vi "arrange func.vi"(10 "input Parameter":T2={"input COP of ACs"=3.0, "input setDay Temp"=22.0, "input setNight Temp."=20.0}, 11 "input envTemp. & elecFee":cluster{"Temp.":dbl[], "elecFee":dbl[]}={"Temp."=[29.6, 26.5, 26.8, 26.8, 26.5, 26.9, 27.8, 28.5, 26.3, 30.1, 33.3, 33.4, 33.9, 32.2, 32.7, 32.7, 32.4, 31.5, 30.5, 29.7, 28.3, 28.2, 27.9, 27.5], "elecFee"=[2.2, 2.2, 2.2, 2.2, 2.2, 2.2, 2.2, 2.2, 3.5, 3.5, 3.5, 3.5, 3.5, 3.5, 3.5, 3.5, 3.5, 3.5, 3.5, 3.5, 3.5, 3.5, 2.2, 2.2]}) -> (0 "Outcome Total elecFee":dbl[](array[numeric]), 3 "OUTCOME":T1(array[cluster]))   [LabVIEW 2014]
panel:
  in  "group 3 power consume (W)":dbl format="%#_13g"
  in  "group 3 Lightening period (h)":i32
  in  "group 2 power consume (W)":dbl format="%#_13g"
  in  "group 2 Lightening period (h)":i32
  in  "group 1 power consume (W)":dbl format="%#_13g"
  in  "group 1 Lightening period (h)":i32
  in  "OK":bool
  # "0~1"
  # "1~2"
  # "2~3"
  # "3~4"
  # "4~5"
  # "5~6"
  # "6~7"
  # "7~8"
  # "8~98~9"
  # "9~10"
  # "10~11"
  # "11~12"
  # "12~13"
  # "13~14"
  # "14~15"
  # "15~16"
  # "16~17"
  # "17~18"
  # "18~19"
  # "19~20"
  # "21~21"
  # "21~22"
  # "22~23"
  # "23~24"
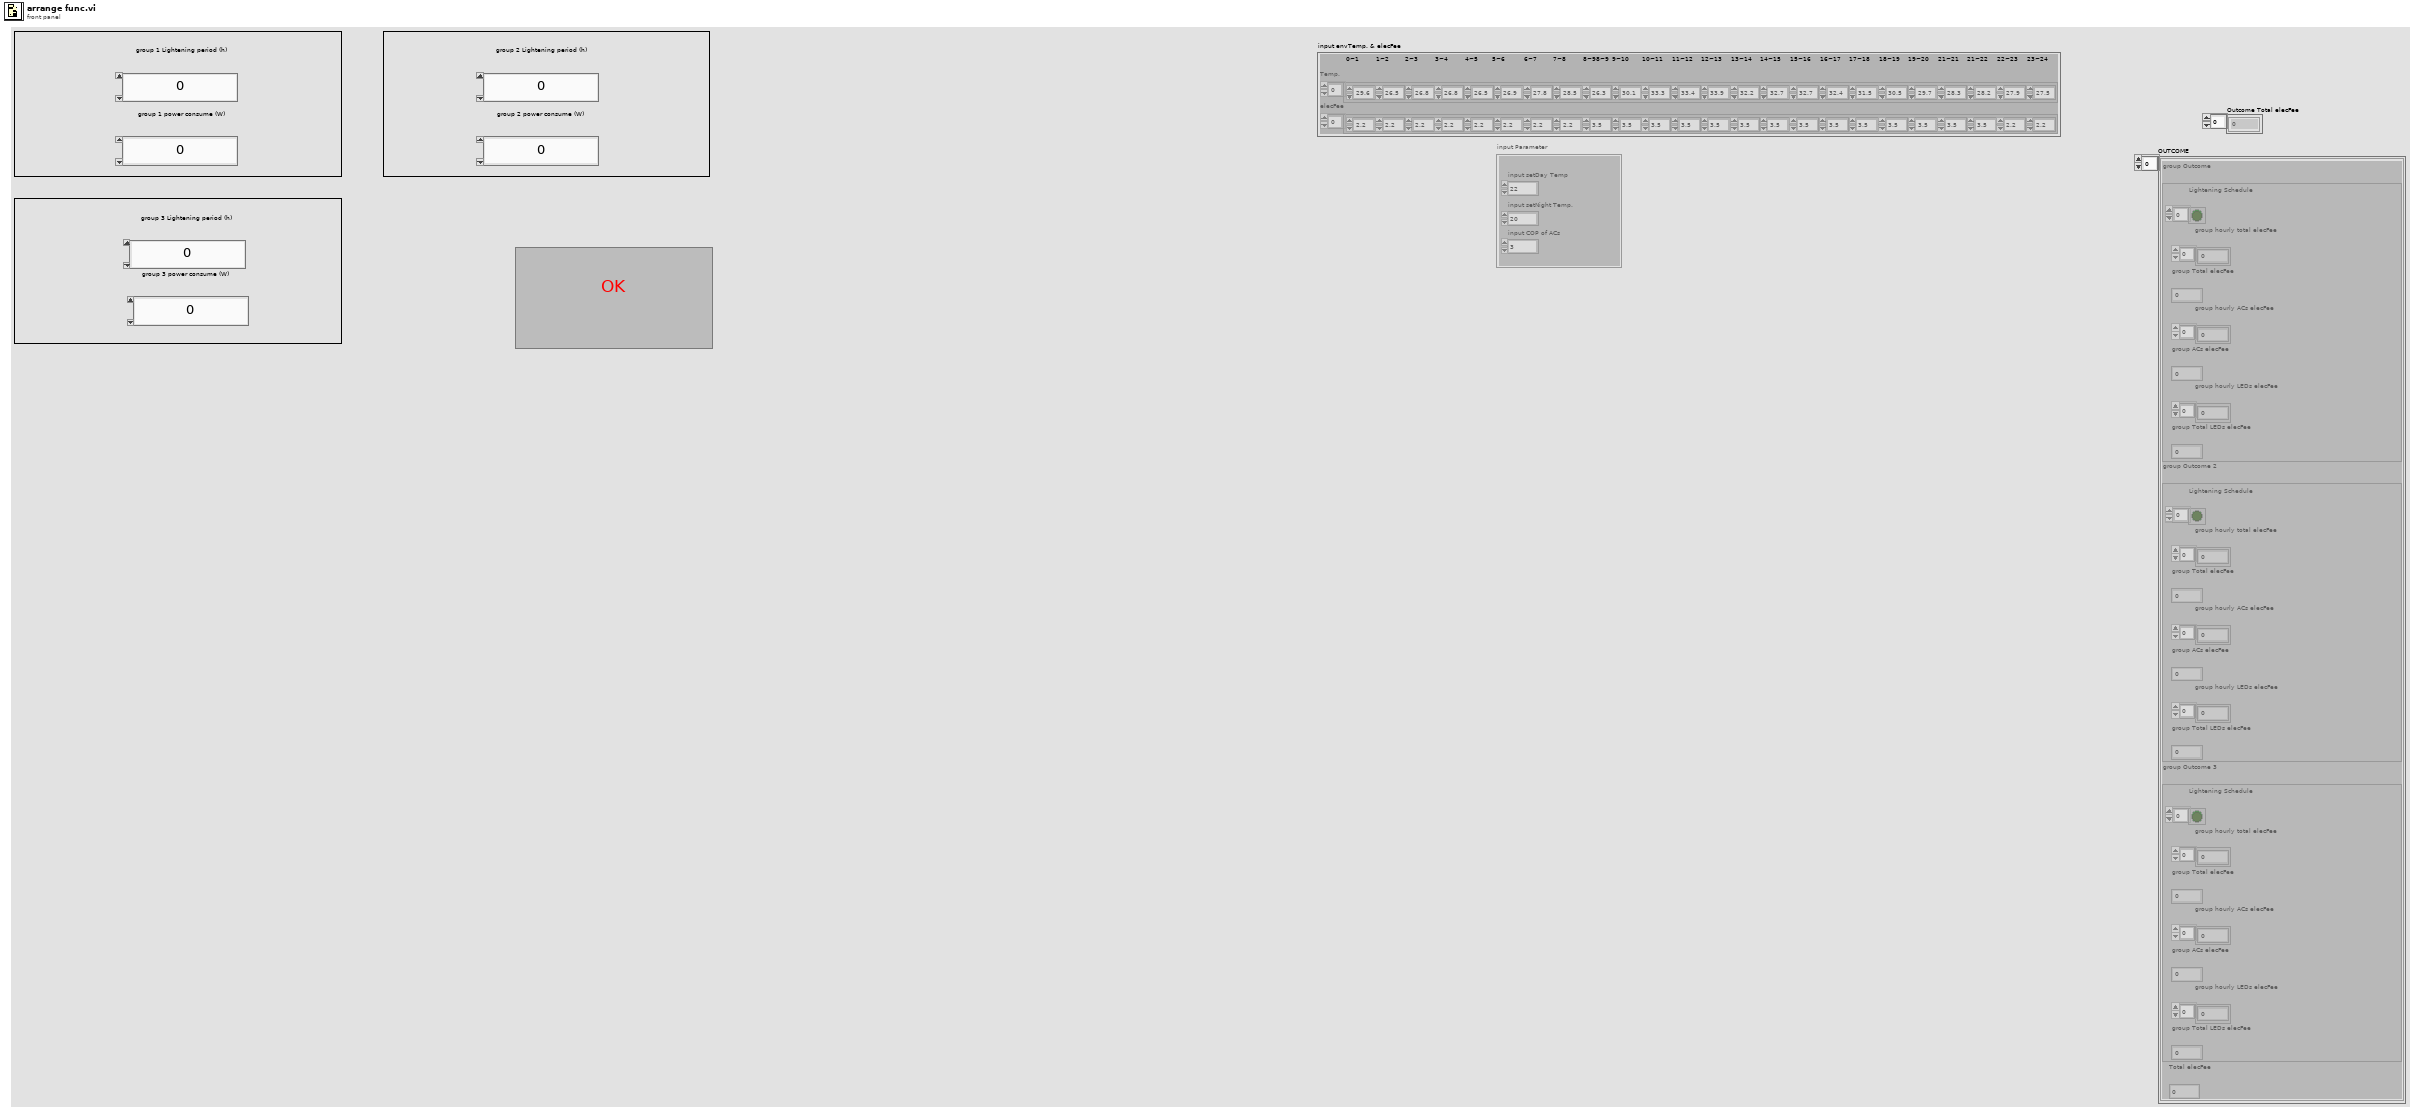
[diagram p1: front panel]
types:
  T1 = cluster{"group Outcome":cluster{"Lightening Schedule":bool[], "group hourly total elecFee":dbl[], "group Total elecFee":dbl, "group hourly ACs elecFee":dbl[], "group ACs elecFee":dbl, "group hourly LEDs elecFee":dbl[], "group Total LEDs elecFee":dbl}, "group Outcome 2":cluster{"Lightening Schedule":bool[], "group hourly total elecFee":dbl[], "group Total elecFee":dbl, "group hourly ACs elecFee":dbl[], "group ACs elecFee":dbl, "group hourly LEDs elecFee":dbl[], "group Total LEDs elecFee":dbl}, "group Outcome 3":cluster{"Lightening Schedule":bool[], "group hourly total elecFee":dbl[], "group Total elecFee":dbl, "group hourly ACs elecFee":dbl[], "group ACs elecFee":dbl, "group hourly LEDs elecFee":dbl[], "group Total LEDs elecFee":dbl}, "Total elecFee":dbl}[]
  T2 = cluster{"input COP of ACs":dbl, "input setDay Temp":dbl, "input setNight Temp.":dbl}
  T3 = cluster{"group Outcome":cluster{"Lightening Schedule":bool[], "group hourly total elecFee":dbl[], "group Total elecFee":dbl, "group hourly ACs elecFee":dbl[], "group ACs elecFee":dbl, "group hourly LEDs elecFee":dbl[], "group Total LEDs elecFee":dbl}, "group Outcome 2":cluster{"Lightening Schedule":bool[], "group hourly total elecFee":dbl[], "group Total elecFee":dbl, "group hourly ACs elecFee":dbl[], "group ACs elecFee":dbl, "group hourly LEDs elecFee":dbl[], "group Total LEDs elecFee":dbl}, "group Outcome 3":cluster{"Lightening Schedule":bool[], "group hourly total elecFee":dbl[], "group Total elecFee":dbl, "group hourly ACs elecFee":dbl[], "group ACs elecFee":dbl, "group hourly LEDs elecFee":dbl[], "group Total LEDs elecFee":dbl}, "Total elecFee":dbl}
  T4 = cluster{"Lightening Schedule":bool[], "group hourly total elecFee":dbl[], "group Total elecFee":dbl, "group hourly ACs elecFee":dbl[], "group ACs elecFee":dbl, "group hourly LEDs elecFee":dbl[], "group Total LEDs elecFee":dbl}
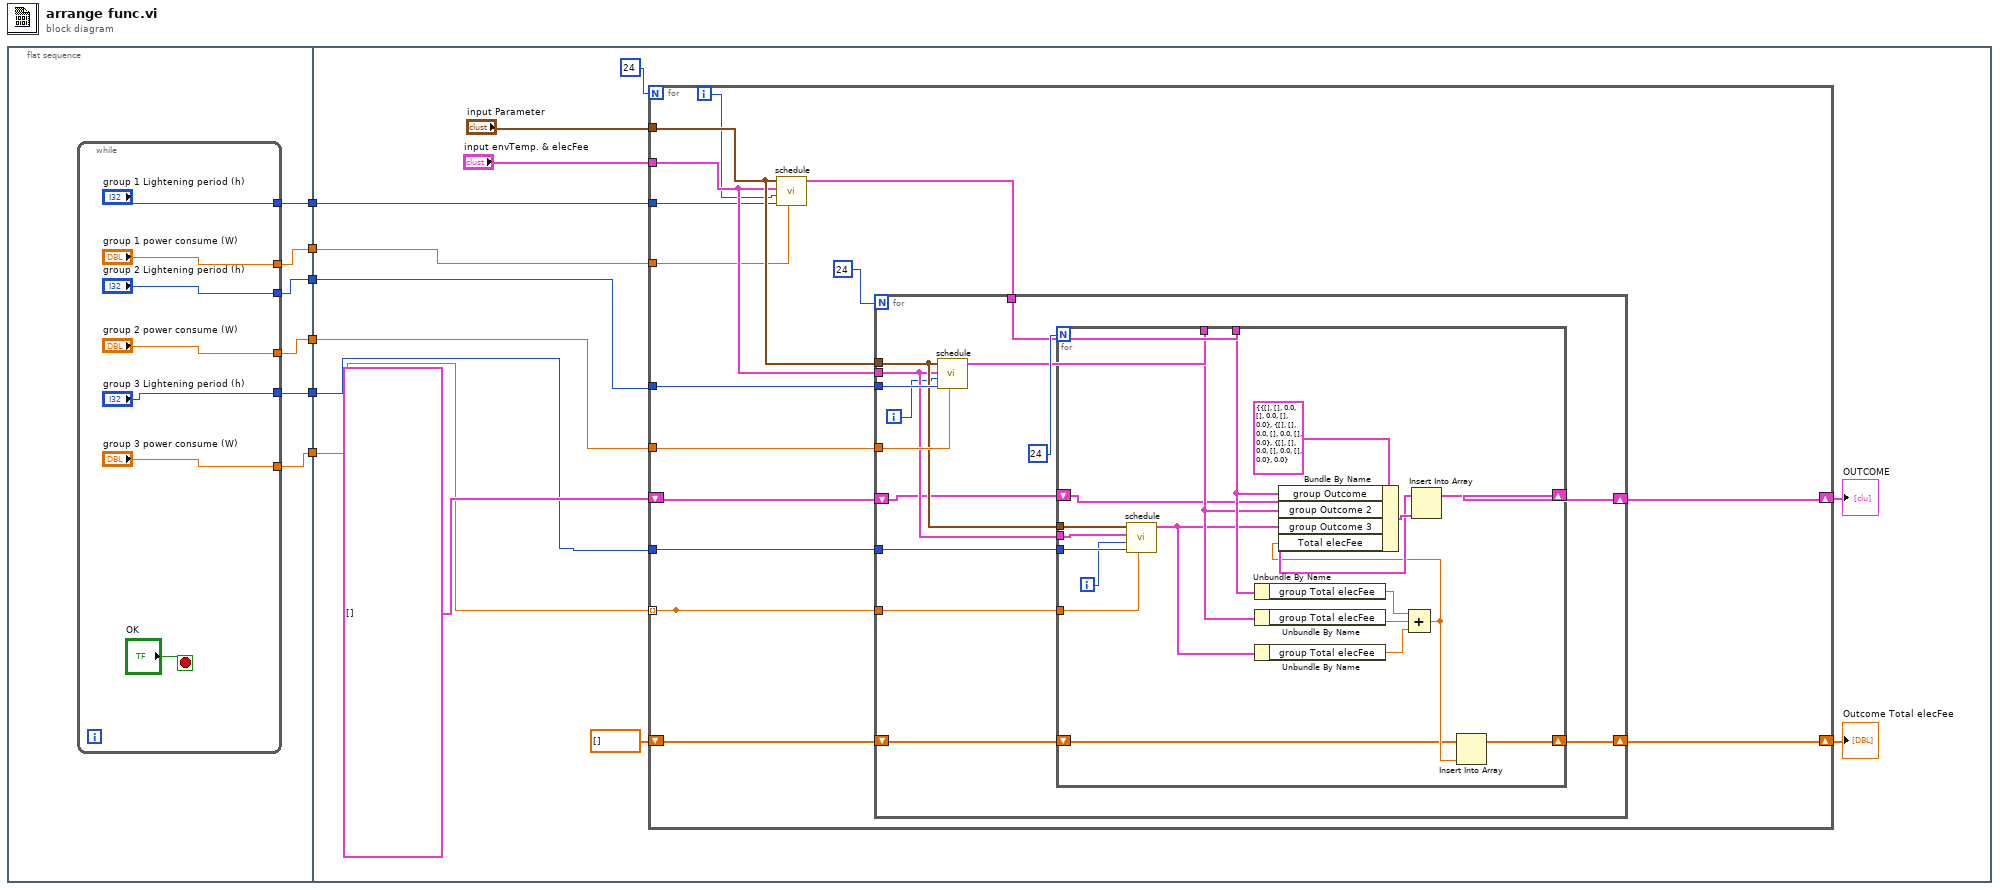
[diagram p0: block diagram]
diagram:
  n1 = flat-sequence {
    tunnel: [w12] -> w6
    tunnel: [w11] -> w5
    tunnel: [w10] -> w4
    tunnel: [w9] -> w3
    tunnel: [w8] -> w2
    tunnel: [w7] -> w1
    tunnel: w6 -> [w26]
    tunnel: w5 -> [w25]
    tunnel: w4 -> [w23]
    tunnel: w3 -> [w22]
    tunnel: w2 -> [w21]
    tunnel: w1 -> [w20]
    frame #0 {
      n2 = while {
        tunnel: ["group 1 Lightening period (h)"] -> w12
        tunnel: ["group 1 power consume (W)"] -> w11
        tunnel: ["group 2 Lightening period (h)"] -> w10
        tunnel: ["group 2 power consume (W)"] -> w9
        tunnel: ["group 3 Lightening period (h)"] -> w8
        tunnel: ["group 3 power consume (W)"] -> w7
        stop <- "OK" stop-if-true
      }
    }
    frame #1 {
      n3 = for {
        N: 24 -> [_]
        tunnel: "input Parameter" -> [w46]
        tunnel: "input envTemp. & elecFee" -> [w45]
        tunnel: w26 -> [w44]
        tunnel: w25 -> [w43]
        tunnel: w23 -> [w42]
        tunnel: w22 -> [w41]
        tunnel: w21 -> [w39]
        tunnel: w20 -> [w38]
        tunnel: [w38] -> _ mode=indexing
        shift-right: [w35] -> w28
        shift-left: T1 [] -> [w36]
        shift-right: [w34] -> w27
        shift-left: dbl[] [] -> [w33]
        i -> [w37]
        n4 = call "schedule.vi"("Lighting Power Consume (W)"=w43, "Lenght of Light Period (hr)"=w44, "Start Time of Light Period"=w37, "input envTemp. & elecFee"=w45, "input Parameter"=w46) -> ("group Outcome"=w40:T4)  [unwired: 6 in]
        n5 = for {
          N: 24 -> [_]
          tunnel: w46 -> [w56]
          tunnel: w45 -> [w55]
          tunnel: w42 -> [w61]
          tunnel: w41 -> [w60]
          tunnel: w40 -> [w58]
          tunnel: w39 -> [w54]
          tunnel: w38 -> [w53]
          shift-right: [w51] -> w35
          shift-left: w36 -> [w50]
          shift-right: [w49] -> w34
          shift-left: w33 -> [w48]
          i -> [w52]
          n6 = call "schedule.vi"("Lighting Power Consume (W)"=w60, "Lenght of Light Period (hr)"=w61, "Start Time of Light Period"=w52, "input envTemp. & elecFee"=w55, "input Parameter"=w56) -> ("group Outcome"=w57:T4)  [unwired: 6 in]
          n7 = for {
            N: 24 -> [_]
            tunnel: w58 -> [w71]
            tunnel: w57 -> [w70]
            tunnel: w56 -> [w79]
            tunnel: w55 -> [w78]
            tunnel: w54 -> [w77]
            tunnel: w53 -> [w76]
            shift-right: [w67] -> w51
            shift-left: w50 -> [w66]
            shift-right: [w64] -> w49
            shift-left: w48 -> [w63]
            i -> [w75]
            n8 = call "schedule.vi"("Lighting Power Consume (W)"=w76, "Lenght of Light Period (hr)"=w77, "Start Time of Light Period"=w75, "input envTemp. & elecFee"=w78, "input Parameter"=w79) -> ("group Outcome"=w69:T4)  [unwired: 6 in]
            n9 = Unbundle By Name(w71) -> ("group Total elecFee"=w74:dbl)
            n10 = Unbundle By Name(w70) -> ("group Total elecFee"=w73:dbl)
            n11 = Unbundle By Name(w69) -> ("group Total elecFee"=w72:dbl)
            n12 = Compound Arithmetic op=ADD(w74, w73, w72) -> (w65:dbl)
            n13 = Bundle By Name(cluster=T3 {"group Outcome"={"Lightening Schedule"=[], "group hourly total elecFee"=[], "group Total elecFee"=0.0, "group hourly ACs elecFee"=[], "group ACs elecFee"=0.0, "group hourly LEDs elecFee"=[], "group Total LEDs elecFee"=0.0}, "group Outcome 2"={"Lightening Schedule"=[], "group hourly total elecFee"=[], "group Total elecFee"=0.0, "group hourly ACs elecFee"=[], "group ACs elecFee"=0.0, "group hourly LEDs elecFee"=[], "group Total LEDs elecFee"=0.0}, "group Outcome 3"={"Lightening Schedule"=[], "group hourly total elecFee"=[], "group Total elecFee"=0.0, "group hourly ACs elecFee"=[], "group ACs elecFee"=0.0, "group hourly LEDs elecFee"=[], "group Total LEDs elecFee"=0.0}, "Total elecFee"=0.0} ("Cluster"), "group Outcome"=w71, "group Outcome 2"=w70, "group Outcome 3"=w69, "Total elecFee"=w65) -> (w68:T3)
            n14 = Insert Into Array(array=w66, new element=w68) -> (w67:T1)  [unwired: 1 in]
            n15 = Insert Into Array(array=w63, new element=w65) -> (w64:dbl[])  [unwired: 1 in]
          }
        }
      }
      "OUTCOME" <- w28
      "Outcome Total elecFee" <- w27
    }
  }
